vi "ThreadCfg - Read RxPkt Config.vi"(8 "error in (no error)":errorcluster, 11 "Node Ptr In":T4 format="%.0x") -> (0 "error out":errorcluster, 2 "threadOptions":T1 {"pclDecimation" max=16 step=1; "loopPeriod" max=16 step=1; "targetPriority" min=-2 max=16 step=1; "targetProcessor" min=-2 max=16 step=1}, 3 "Node Ptr Out":T4 format="%.0x")   [LabVIEW 2023, in "UDP-Custom-Device System Explorer.lvlib"]
uses:
  UDP-Custom-Device System Explorer.lvlib
  <vilib>/NI VeriStand/Custom Device API/Custom Device Item Ref.ctl
  Types/Threading/Thread Configuration.ctl
  Types/Threading/Thread Sync Reference.ctl
  Shared/Types/Shared - Thread Management.ctl
  Property Accessors/Shared Packet Accessors.lvlib
  Shared/UDP-Custom-Device Shared.lvlib
  <vilib>/NI VeriStand/Custom Device API/Custom Device API.lvlib
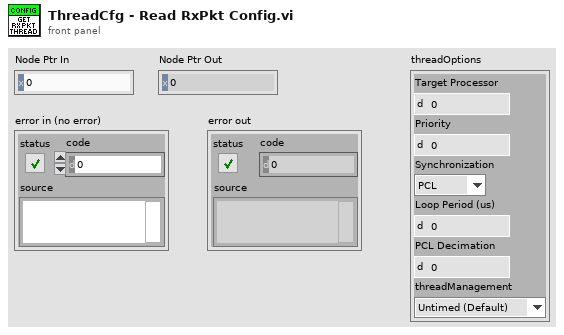
[diagram p1: front panel]
types:
  T1 = typedef "UDP-Custom-Device System Explorer.lvlib/Thread Configuration.ctl" = cluster{"targetProcessor":i8, "targetPriority":i16, "Synchronization":T2, "loopPeriod":u32, "pclDecimation":u16, "threadManagement":T3}
  T2 = typedef "UDP-Custom-Device System Explorer.lvlib/Thread Sync Reference.ctl" = enum16{"PCL", "Async"}
  T3 = typedef "UDP-Custom-Device Shared.lvlib/Shared - Thread Management.ctl" = enum16{"Untimed (Default)", "Timed (High Priority)"}
  T4 = typedef "Custom Device API.lvlib/Custom Device Item Ref.ctl" = u64
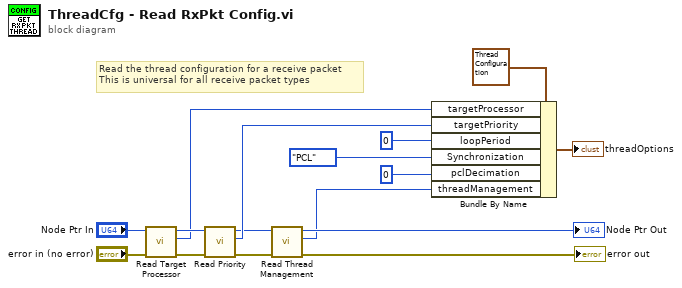
[diagram p0: block diagram]
diagram:
  # "Read the thread configuration for a receive packet\nThis is universal for all receive packet types"
  n1 = call "Read Target Processor.vi"("error in (no error)"="error in (no error)", "Node Ptr"="Node Ptr In") -> ("error out"=w13:errorcluster, "targetProcessor"=w9:i8, "Node Ptr out"=w14:T4)  [unwired: 7 in]
  n2 = call "Read Priority.vi"("error in (no error)"=w13, "Node Ptr"=w14) -> ("error out"=w3:errorcluster, "targetPriority"=w10:i16, "Node Ptr out"=w5:T4)  [unwired: 7 in]
  n3 = call "Read Thread Management.vi"("error in (no error)"=w3, "Node Ptr"=w5) -> ("error out"=→"error out":errorcluster, "Thread Management"=w1:T3, "Node Ptr out"=→"Node Ptr Out":T4)  [unwired: 7 in]
  n4 = Bundle By Name(cluster=T1 {"targetProcessor"=0, "targetPriority"=0, "Synchronization"=enum."PCL", "loopPeriod"=0, "pclDecimation"=0, "threadManagement"=enum."Untimed (Default)"} ("threadOptions"), "targetProcessor"=w9, "targetPriority"=w10, "loopPeriod"=0, "Synchronization"=Thread_Sync_Reference."PCL", "pclDecimation"=u16 0, "threadManagement"=w1) -> (→"threadOptions":T1)
